vi "Capteur avec Modbus.vi"() -> ()   [LabVIEW 2013]
uses:
  <instrlib>/K_S30c_VISA/K_S30c_VISA.lvlib
panel:
  in  "Port":refnum<visa-resource-name>="COM1"
  in  "Baudrate":enum16{"9600", "115200"}(ring)
  in  "timeout":u32=50
  in  "Open Com":bool
  in  "Address":u8=250
  in  "Channel":enum16{"CH0", "P1", "P2", "T", "TOB1", "TOB2"}(ring)=enum."P1"
  out "Value":sgl(graph)
  out "error":errorcluster
  in  "Online":bool
  in  "Stop":bool
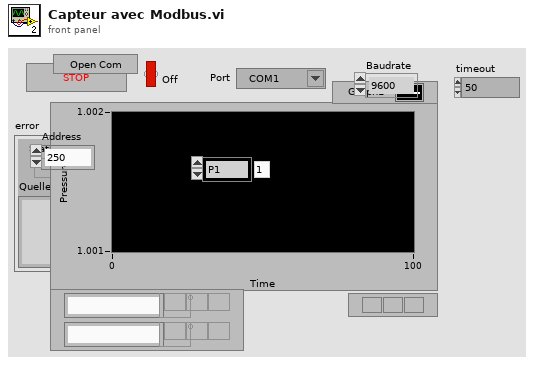
[diagram p1: front panel]
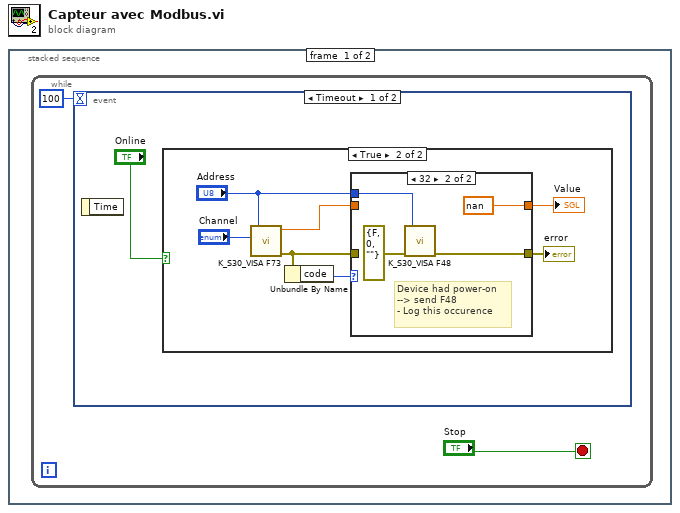
[diagram p0: block diagram]
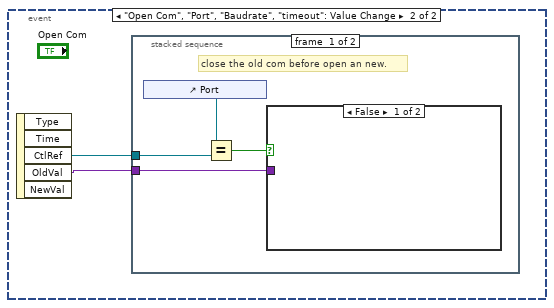
[diagram p4: hidden frame]
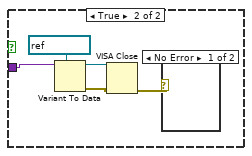
[diagram p5: hidden frame]
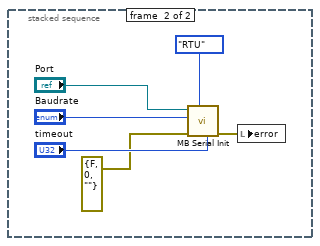
[diagram p7: hidden frame]
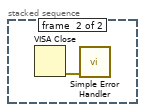
[diagram p8: hidden frame]
diagram:
  n1 = stacked-sequence {
    frame #0 {
      n2 = while {
        stop <- "Stop" stop-if-true
        n3 = event shown="[0] Timeout" {
          selector: _ -> [_ _]
          dyn-events: _ -> [_ _]
          timeout: 100 -> [_ _]
          event Timeout {
            n4 = event-data() -> ()  [unwired: 1 in, 1 out]
            n5 = case shown="True" "Online" {
              frame False {
              }
              frame True {
                n6 = call <instrlib>:"K_S30_VISA F73.vi"("Channel"="Channel", "Address"="Address") -> ("error out"=w7:errorcluster, "Value"=w6:sgl)  [unwired: 3 in, 1 out]
                n7 = Unbundle By Name(w7) -> ("code"=w9:i32)
                n8 = case shown="32" w9 {
                  tunnel: "Address" -> [_ w15]
                  tunnel: w7 -> [w11 _]
                  tunnel: w6 -> [w12 _]
                  tunnel: [w12 sgl nan] -> w5
                  tunnel: [w11 w13] -> w4
                  frame 0, Default {
                  }
                  frame 32 {
                    # "Device had power-on\n--> send F48\n- Log this occurence"
                    n9 = call <instrlib>:"K_S30_VISA F48.vi"("error in"=errorcluster {"status"=FALSE, "code"=0, "source"=""}, "Address"=w15) -> ("error out"=w13:errorcluster)  [unwired: 3 in, 2 out]
                  }
                }
                "Value" <- w5
                "error" <- w4
              }
            }
          }
          event "Open Com", "Port", "Baudrate", "timeout": Value Change {
            n10 = event-data() -> ("CtlRef"=w18:refnum<vi>, "OldVal"=w17:variant)  [unwired: 1 in, 3 out]
            n11 = stacked-sequence {
              tunnel: w18 -> [w20 _]
              tunnel: w17 -> [w21 _]
              frame #0 {
                # "close the old com before open an new."
                n12 = control-ref of="Port"() -> (w19:refnum<vi>)
                n13 = Equal?(x=w19, y=w20) -> (x = y?=w22:bool)
                n14 = case shown="False" w22 {
                  tunnel: w21 -> [_ w27]
                  frame False {
                  }
                  frame True {
                    n15 = Variant To Data(type=refnum<visa-resource-name> "COM1" ("VISA resource name"), Variant=w27) -> (data=w25:refnum<visa-resource-name>, error out=w24:errorcluster)  [unwired: 1 in]
                    n16 = VISA Close(VISA resource name=w25, error in (no error)=w24) -> (error out=w23:errorcluster)
                    n17 = case shown="No Error" w23 {
                      frame No Error {
                      }
                      frame Error {
                      }
                    }
                  }
                }
              }
              frame #1 {
                n18 = call <vilib>:"MB Serial Init.vi"("Timeout"="timeout", "Mode"=enum16{"RTU"}."RTU", "error in (no error)"=errorcluster {"status"=FALSE, "code"=0, "source"=""}, "Baud Rate"="Baudrate", "VISA resource name"="Port") -> ("error out"=w30:errorcluster)  [unwired: 5 in, 1 out]
                n19 = local write "error"(w30) -> ()
              }
            }
          }
        }
      }
    }
    frame #1 {
      n20 = VISA Close() -> (error out=w34:errorcluster)  [unwired: 2 in]
      n21 = call <vilib>:"Simple Error Handler.vi"("error in (no error)"=w34) -> ()  [unwired: 1 in, 8 out]
    }
  }
